vi "FGV_TSE_Status.vi"(2 "TSE_Status_In":T1={"Return Code"=0, "Message"="", "error in (no error)"={"status"=FALSE, "code"=0, "source"=""}, "Program State"=enum."Ön Yükleme Tamam", "Test A. Suresi"=0}, 3 "Operation":enum16{"Get", "Set"}(ring)) -> (1 "TSE_Status_Out":T1={"Return Code"=0, "Message"="", "error in (no error)"={"status"=FALSE, "code"=0, "source"=""}, "Program State"=enum."Ön Yükleme Tamam", "Test A. Suresi"=0})   [LabVIEW 2014]
uses:
  CustomControls/TSE_Status.ctl
  CustomControls/Program_States.ctl
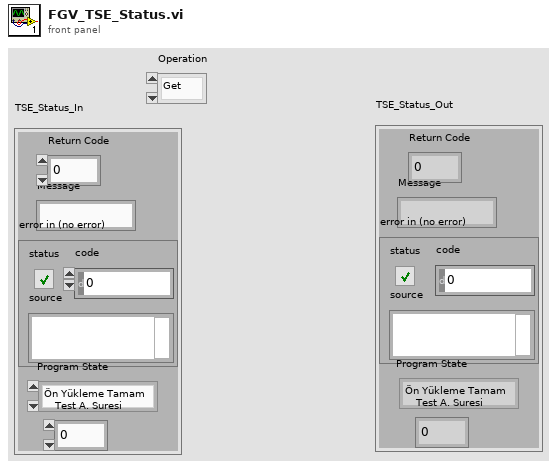
[diagram p1: front panel]
types:
  T1 = typedef "TSE_Status.ctl" = cluster{"Return Code":i32, "Message":string, "error in (no error)":errorcluster, "Program State":T2, "Test A. Suresi":u32}
  T2 = typedef "Program_States.ctl" = enum16{"Ön Yükleme", "TSE Baslat", "Kalibratöre Baglan", "Kalibratörü Baslat", "Ön Yükleme Tamam", "Frekans Testi", "Gerilim Testi", "Akim Testi", "Aktif Guc Testi", "Reaktif Guc Testi", "AC Akim Harmonik Testi", "AC Gerilim Harmonik Testi", "Flicker Testi", "Rapor Cikarma", "Yeniden Başlat", "Bekleme", "Durdur"}
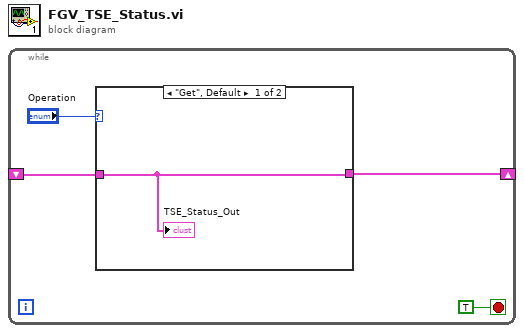
[diagram p0: block diagram]
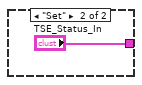
[diagram p2: hidden frame]
diagram:
  n1 = while {
    shift-right: [w2] -> _
    shift-left: _ -> [w1]
    stop <- TRUE stop-if-true
    n2 = case shown="\"Get\", Default" "Operation" {
      tunnel: [w5 "TSE_Status_In"] -> w2
      tunnel: w1 -> [w5 _]
      frame "Get", Default {
        "TSE_Status_Out" <- w5
      }
      frame "Set" {
      }
    }
  }
